vi "SetAlpha.vi"(8 "error in (no error)":errorcluster, 10 "Alpha":u8, 11 "ColorRGBA in":refnum<class "ColorRGBA.lvclass">) -> (0 "error out":errorcluster, 3 "ColorRGBA out":refnum<class "ColorRGBA.lvclass">)   [LabVIEW 2021, in "Picture2D.lvlib" / "ColorRGBA.lvclass"]
uses:
  ColorRGBA.lvclass
  ColorRGBA.lvclass/ColorRGBA.ctl
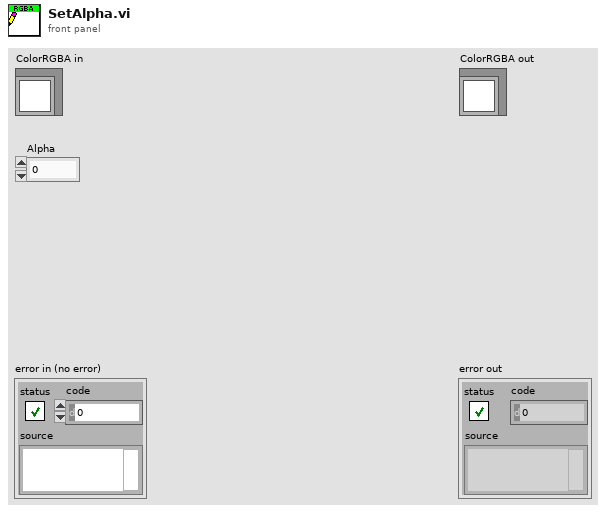
[diagram p1: front panel]
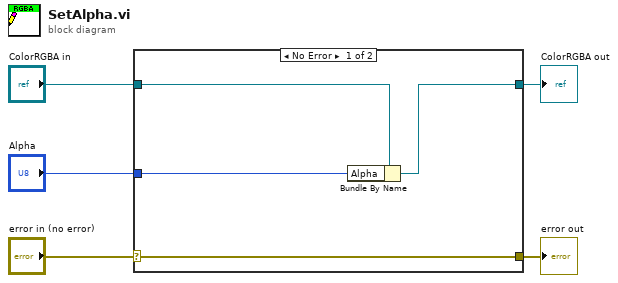
[diagram p0: block diagram]
diagram:
  n1 = case shown="No Error" "error in (no error)" {
    selector: "error in (no error)" -> [w9 w10]
    tunnel: [w9 w10] -> w4
    tunnel: [w7 w11] -> w2
    tunnel: "ColorRGBA in" -> [w8 w11]
    tunnel: "Alpha" -> [w6 _]
    frame No Error {
      n2 = Bundle By Name(cluster=w8, "Alpha"=w6) -> (w7:refnum<class "ColorRGBA.lvclass">)
    }
    frame Error {
    }
  }
  "error out" <- w4
  "ColorRGBA out" <- w2
